vi "ScrubNudge.vi"   [LabVIEW 2014]
uses:
  <vilib>/Rock Robotics/WPI/Joystick/WPI_JoystickGetSetRefNum.vi
  Gantry/GantryGlobals.vi
  AutomationGlobals.vi
types:
  T1 = typedef "WPI_JoystickDevRef.ctl" = cluster{"Device":T2}
  T2 = typedef "WPI_JoystickDeviceEnum.ctl" = enum16{"USB 0", "USB 1", "USB 2", "USB 3", "USB 4", "USB 5"}
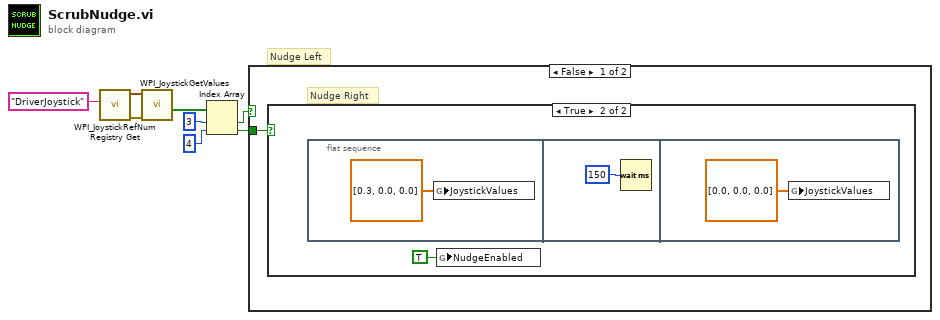
[diagram p0: block diagram]
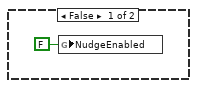
[diagram p2: hidden frame]
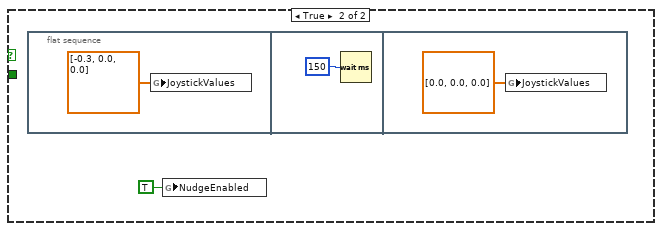
[diagram p3: hidden frame]
diagram:
  # "Nudge Left"
  n1 = call <vilib>:"WPI_JoystickRefNum Registry Get.vi"("refnum name"="DriverJoystick") -> ("error out"=w8:errorcluster, "JoystickDevRef"=w7:T1)  [unwired: 9 in]
  n2 = call <vilib>:"WPI_JoystickGetValues.vi"("error in (no error)"=w8, "JoystickDevRef"=w7) -> ("Buttons"=w5:bool[])  [unwired: 5 in, 4 out]
  n3 = Index Array(array=w5, index #1=3 ("index"), index #2=4 ("index")) -> (element #1=w2:bool, element #2=w1:bool)
  n4 = case shown="False" w2 {
    tunnel: w1 -> [w9 _]
    frame False {
      # "Nudge Right"
      n5 = case shown="True" w9 {
        frame False {
          n6 = global write "GantryGlobals.vi" "NudgeEnabled"(FALSE ("NudgeEnabled")) -> ()
        }
        frame True {
          n7 = flat-sequence {
            frame #0 {
              n8 = global write "AutomationGlobals.vi" "JoystickValues"(dbl[] [0.3, 0.0, 0.0] ("JoystickValues")) -> ()
            }
            frame #1 {
              n9 = Wait (ms)(milliseconds to wait=u32 150) -> ()  [unwired: 1 out]
            }
            frame #2 {
              n10 = global write "AutomationGlobals.vi" "JoystickValues"(dbl[] [0.0, 0.0, 0.0] ("JoystickValues")) -> ()
            }
          }
          n11 = global write "GantryGlobals.vi" "NudgeEnabled"(TRUE ("NudgeEnabled")) -> ()
        }
      }
    }
    frame True {
      n12 = flat-sequence {
        frame #0 {
          n13 = global write "AutomationGlobals.vi" "JoystickValues"(dbl[] [-0.3, 0.0, 0.0] ("JoystickValues")) -> ()
        }
        frame #1 {
          n14 = Wait (ms)(milliseconds to wait=u32 150) -> ()  [unwired: 1 out]
        }
        frame #2 {
          n15 = global write "AutomationGlobals.vi" "JoystickValues"(dbl[] [0.0, 0.0, 0.0] ("JoystickValues")) -> ()
        }
      }
      n16 = global write "GantryGlobals.vi" "NudgeEnabled"(TRUE ("NudgeEnabled")) -> ()
    }
  }
